vi "send_string_01.vi"(0 "connection ID":refnum<k5>, 1 "String flag (i s)":string, 2 "Input string":string, 3 "error out":errorcluster, 4 "Reader ID":string) -> (5 "connection ID 2":refnum<k5>, 6 "answer":string, 7 "error IO":errorcluster)   [LabVIEW 2010]
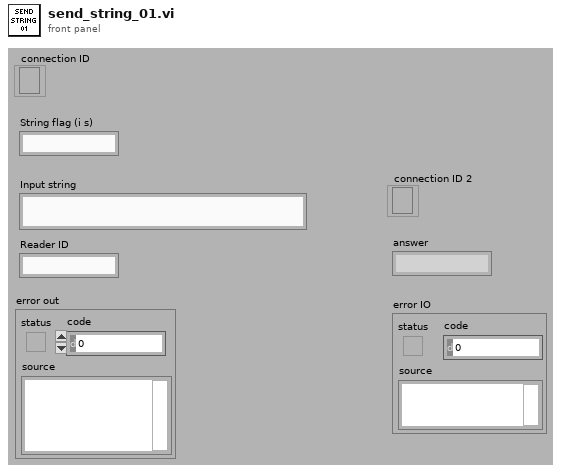
[diagram p1: front panel]
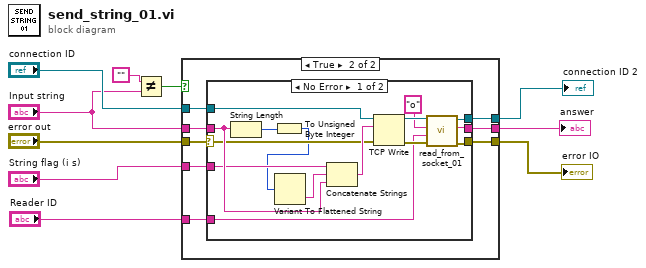
[diagram p0: block diagram]
diagram:
  n1 = Not Equal?(x="", y="Input string") -> (x != y?=w3:bool)
  n2 = case shown="True" w3 {
    tunnel: [w12 w21] -> w10
    tunnel: "Input string" -> [w12 w20]
    tunnel: "error out" -> [w11 w19]
    tunnel: "connection ID" -> [w13 w18]
    tunnel: "Reader ID" -> [_ w17]
    tunnel: [w13 w16] -> w6
    tunnel: [w11 w15] -> w5
    tunnel: "String flag (i s)" -> [_ w14]
    frame False {
    }
    frame True {
      n3 = case shown="No Error" w19 {
        selector: w19 -> [w24 w38]
        tunnel: [w30 w38] -> w15
        tunnel: w18 -> [w32 w37]
        tunnel: [w31 w37] -> w16
        tunnel: [w29 _] -> w21
        tunnel: w20 -> [w27 _]
        tunnel: w17 -> [w26 _]
        tunnel: w14 -> [w25 _]
        frame No Error {
          n4 = String Length(string=w27) -> (length=w23:i32)
          n5 = To Unsigned Byte Integer(number=w23) -> (unsigned 8bit integer=w22:u8)
          n6 = Variant To Flattened String(Variant=w22) -> (data string=w36:string)  [unwired: 1 out]
          n7 = Concatenate Strings(w25, w36, w27) -> (w28:string)
          n8 = TCP Write(connection ID=w32, data in=w28, error in (no error)=w24) -> (connection ID out=w34:refnum<k5>, error out=w35:errorcluster)  [unwired: 1 in, 1 out]
          n9 = call "read_from_socket_01.vi"("error out"=w35, "Reader ID"=w26, "correct answer"="o", "In connection ID"=w34) -> ("warning out"=w30:errorcluster, "answer"=w29:string, "Out connection ID"=w31:refnum<k5>)  [unwired: 1 in]
        }
        frame Error {
        }
      }
    }
  }
  "answer" <- w10
  "connection ID 2" <- w6
  "error IO" <- w5
